vi "Storage Classes.vi"() -> ()   [LabVIEW 2020]
panel:
  in  "i64":i64
  in  "u64":u64
  in  "i32":i32
  in  "u32":u32
  in  "i16":i16
  in  "u16":u16
  in  "i8":i8
  in  "u8":u8
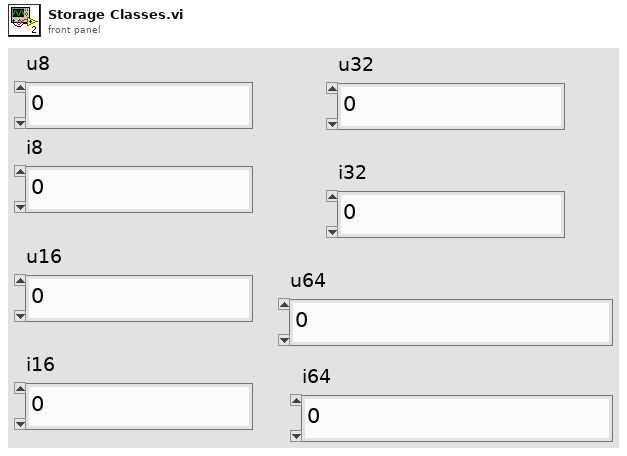
[diagram p1: front panel]
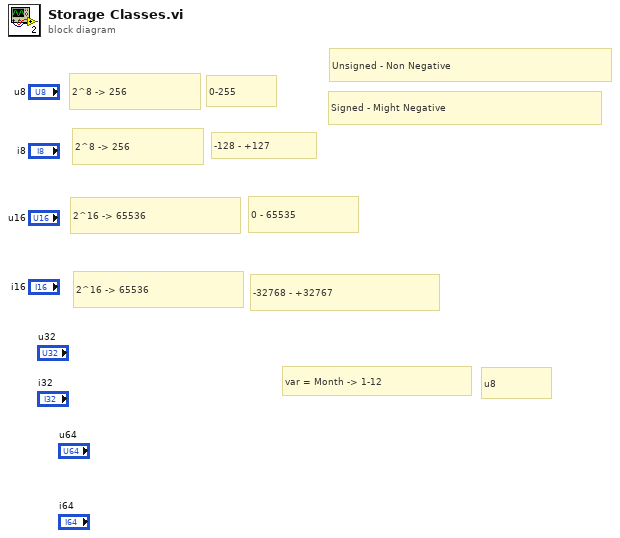
[diagram p0: block diagram]
diagram:
  # "u8"
  # "var = Month -> 1-12"
  # "-32768 - +32767"
  # "2^16 -> 65536"
  # "0 - 65535"
  # "2^16 -> 65536"
  # "-128 - +127"
  # "2^8 -> 256"
  # "Signed - Might Negative"
  # "Unsigned - Non Negative"
  # "0-255"
  # "2^8 -> 256"
